vi "TestAdd.vi"(8 "error in (no error)":errorcluster, 11 "TestCase in":refnum<class "CalculatorTestCase.lvclass">) -> (0 "error out":errorcluster, 3 "TestCase out":refnum<class "CalculatorTestCase.lvclass">)   [LabVIEW 2020, in "CalculatorTestCase.lvclass"]
uses:
  CalculatorTestCase.lvclass
  LabVIEW Data/Calculator/Calculator.lvclass
  <vilib>/addons/_JKI Toolkits/VI Tester/TestCase.llb/TestCase.lvclass
  C:/Program Files (x86)/National Instruments/LabVIEW 2020/vi.lib/addons/_JKI Toolkits/VI Tester/TestCase.llb/TestCase.lvclass
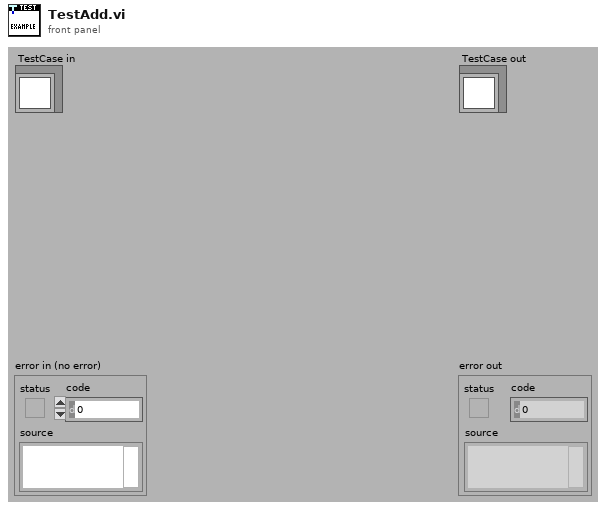
[diagram p1: front panel]
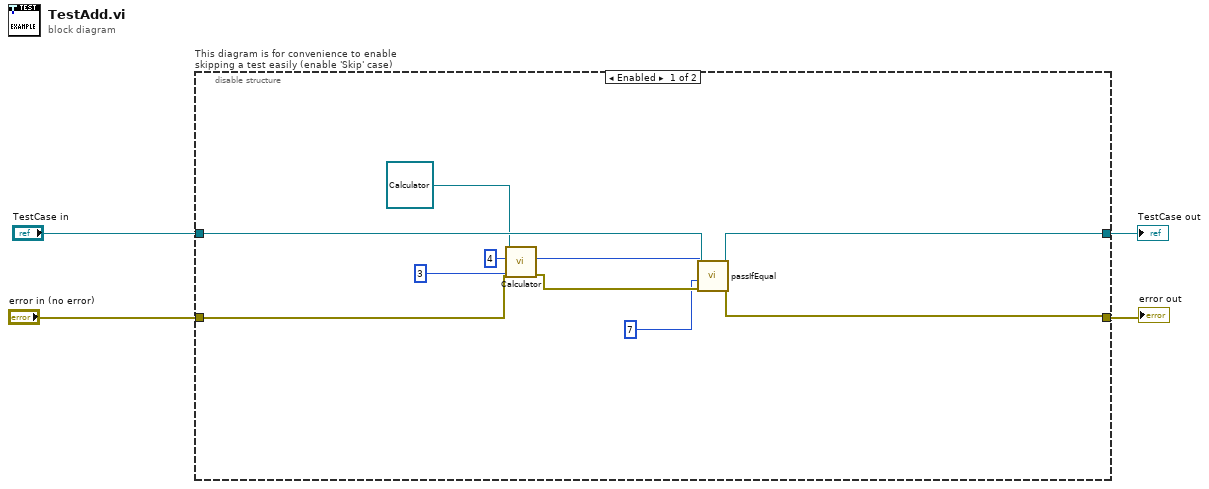
[diagram p0: block diagram]
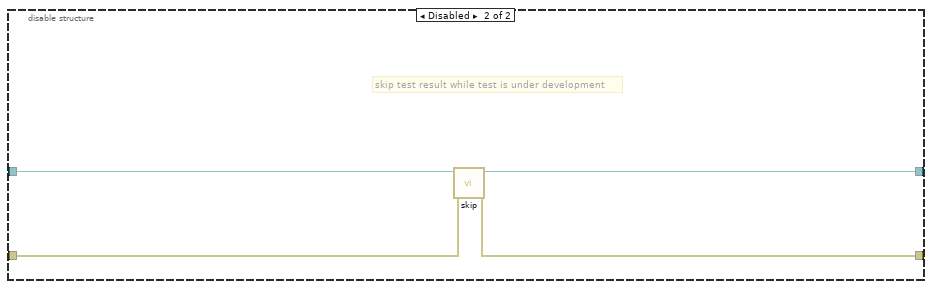
[diagram p2: hidden frame]
diagram:
  n1 = disable-structure "This diagram is for convenience to enable skipping a test easily (enable 'Skip' case)" shown="Enabled" {
    disable-tunnel: "TestCase in" -> [w14 w18]
    disable-tunnel: [w13 w16] -> w1
    disable-tunnel: [w12 w17] -> w3
    disable-tunnel: "error in (no error)" -> [w7 w15]
    frame Enabled {
      n2 = call "Calculator.vi"("error in (no error)"=w7, "Input 2"=3, "Input 1"=4, "Calculator in"=refnum<class "Calculator.lvclass"> refnum) -> ("error out"=w6:errorcluster, "Output"=w11:i32)  [unwired: 5 in, 1 out]
      n3 = call-dynamic "passIfEqual.vi"("error in (no error)"=w6, "y"=7, "x"=w11, "TestCase in"=w14) -> ("error out"=w12:errorcluster, "TestCase out"=w13:refnum<class "CalculatorTestCase.lvclass">)  [unwired: 6 in]
    }
    frame Disabled {
      # "skip test result while test is under development"
      n4 = call <vilib>:"skip.vi"("error in (no error)"=w15, "TestCase in"=w18) -> ("error out"=w17:errorcluster, "TestCase out"=w16:refnum<class "CalculatorTestCase.lvclass">)  [unwired: 8 in]
    }
  }
  "error out" <- w3
  "TestCase out" <- w1
